vi "main file settings panel.vi"() -> ()   [LabVIEW 2013]
panel:
  in  "File Segmenting size (MB)":dbl
  in  "Segment file according to size?":bool
  in  "Channel browser with check boxes":cluster{}
  in  "File Path Control":path
  # "(another panel for File Description and \nfile properties)"
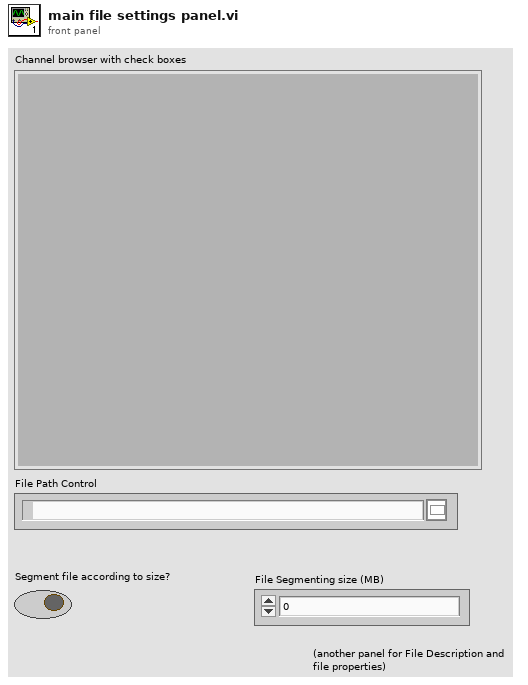
[diagram p1: front panel]
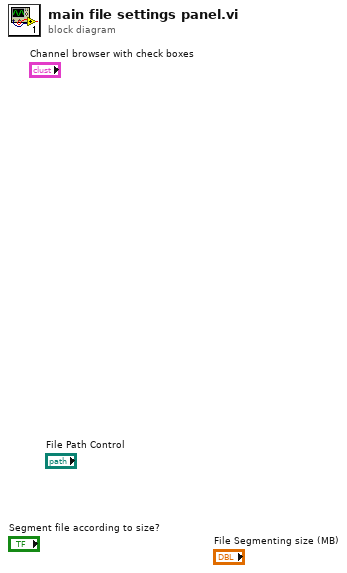
[diagram p0: block diagram]
diagram:
